vi "Main - Get MAC Address.vi"(8 "error in (no error)":errorcluster) -> (0 "error out":errorcluster, 3 "MAC Address":string[](array[string]))   [LabVIEW 2019]
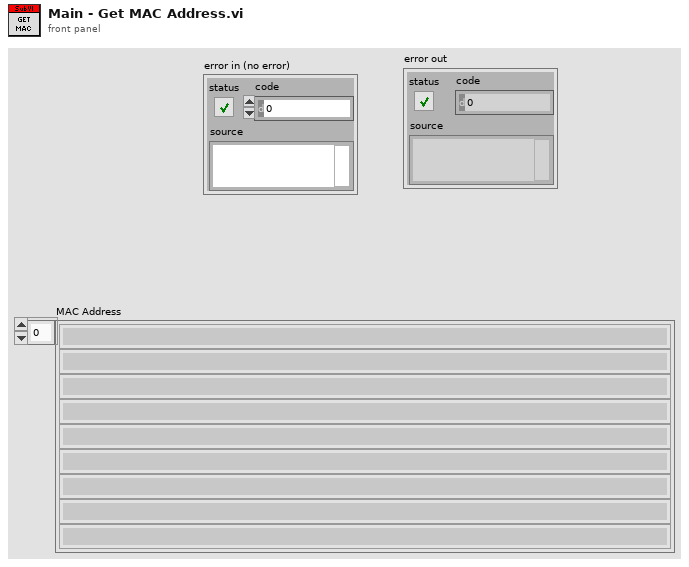
[diagram p1: front panel]
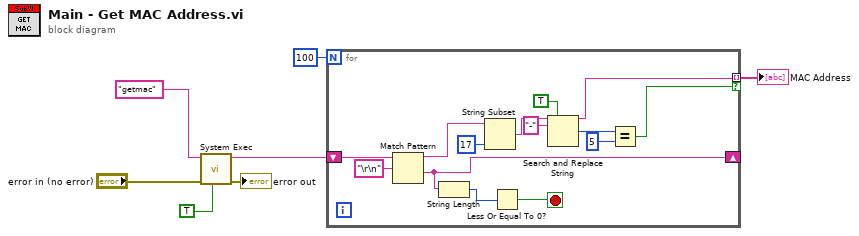
[diagram p0: block diagram]
diagram:
  n1 = call <vilib>:"System Exec.vi"("run minimized? (F)"=TRUE, "error in (no error)"="error in (no error)", "command line"="getmac") -> ("error out"=→"error out":errorcluster, "standard output"=w6:string)  [unwired: 5 in, 2 out]
  n2 = for {
    N: 100 -> [_]
    shift-right: [w19] -> _
    shift-left: w6 -> [w21]
    tunnel: [w8] -> w5 mode=indexing if=w10
    stop <- w17 stop-if-true
    n3 = Match Pattern(string=w21, regular expression="\r\n") -> (before substring=w16:string, after substring=w19:string)  [unwired: 1 in, 2 out]
    n4 = String Length(string=w19) -> (length=w18:i32)
    n5 = String Subset(string=w16, length (rest)=17 ("length (rest)")) -> (substring=w9:string)  [unwired: 1 in]
    n6 = Less Or Equal To 0?(x=w18) -> (x <= 0?=w17:bool)
    n7 = Search and Replace String(replace all?=TRUE ("replace all? (F)"), input string=w9, search string="-") -> (result string=w8:string, number of replacements=w12:i32)  [unwired: 5 in, 2 out]
    n8 = Equal?(x=w12, y=5) -> (x = y?=w10:bool)
  }
  "MAC Address" <- w5
